vi "To Dynamic Signal.vi"(8 "error in (no error)":errorcluster, 11 "Software Lock-in in":refnum<class "Software Lock-in.lvclass">) -> (0 "error out":errorcluster, 1 "Channel names":string[](array[string]), 2 "Signal":dynamicdata(graph), 3 "Software Lock-in out":refnum<class "Software Lock-in.lvclass">, 4 "Time axis":dbl[](array[numeric]), 5 "dt":dbl)   [LabVIEW 2020, in "Software Lock-in.lvclass"]
uses:
  Software Lock-in.lvclass
  C:/GitHub/NHMFL_Core/Libraries/SoftwareLockin/Lock-in Detector/Lock-in Detector.lvclass
  Lock-in Detector/Lock-in Detector.lvclass/Lock-in Detector.ctl
  Software Lock-in.lvclass/Software Lock-in.ctl
  Lock-in Detector/Read Harmonic.vi
  Lock-in Detector/Read Decimation factor.vi
  Lock-in Detector/Read Sample rate.vi
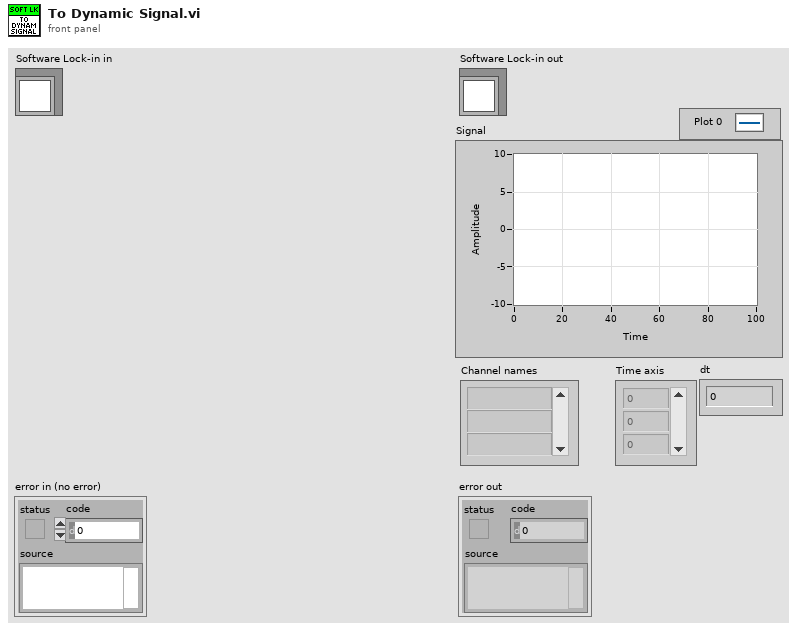
[diagram p1: front panel]
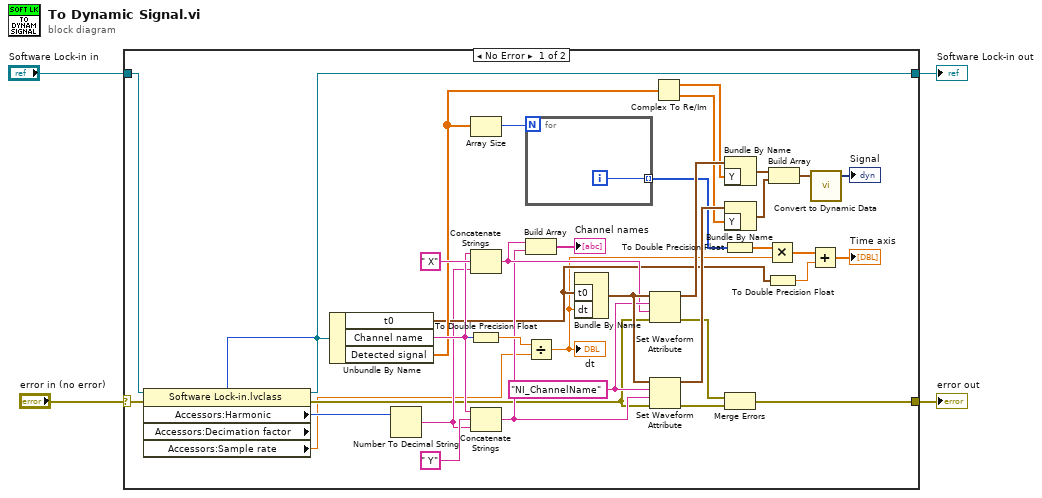
[diagram p0: block diagram]
diagram:
  n1 = case shown="No Error" "error in (no error)" {
    selector: "error in (no error)" -> [w25 w44]
    tunnel: [w24 w44] -> w3
    tunnel: [w8 w43] -> w1
    tunnel: "Software Lock-in in" -> [w9 w43]
    frame No Error {
      w38 = "NI_ChannelName" ("Channel Name")
      n2 = property class="Software Lock-in.lvclass"(reference=w9, error in=w25) -> (reference out=w8:refnum<class "Software Lock-in.lvclass">, error out=w10:errorcluster, "Accessors:Harmonic"=w7:i32, "Accessors:Decimation factor"=w6:i32, "Accessors:Sample rate"=w5:dbl)
      n3 = Unbundle By Name(w8) -> ("t0"=w15:timestamp, "Channel name"=w36:string, "Detected signal"=w20:cdb[])
      n4 = Number To Decimal String(number=w7) -> (decimal integer string=w11:string)  [unwired: 1 in]
      n5 = Array Size(array=w20) -> (size(s)=w19:i32)
      n6 = Concatenate Strings(w36, " X" ("string"), w11) -> (w23:string)
      n7 = To Double Precision Float(number=w6) -> (double precision float=w41:dbl)
      n8 = Concatenate Strings(w36, " Y" ("string"), w11) -> (w22:string)
      n9 = for {
        N: w19 -> [_]
        tunnel: [w42] -> w18 mode=indexing
        i -> [w42]
      }
      n10 = Build Array(w23, w22) -> (→"Channel names":string[])
      n11 = Divide(x=w41, y=w5) -> (x/y=w12:dbl)
      "dt" <- w12
      n12 = Bundle By Name("t0"=w15, "dt"=w12) -> (w39:waveform(dbl))  [unwired: 1 in]
      n13 = Set Waveform Attribute(4:w10, 5:w23, 6:w38, 7:w39) -> (0:w27:errorcluster, 3:w35:waveform(dbl))  [unwired: 1 out]
      n14 = Set Waveform Attribute(4:w10, 5:w22, 6:w38, 7:w39) -> (0:w26:errorcluster, 3:w33:waveform(dbl))  [unwired: 1 out]
      n15 = Complex To Re/Im(x + iy=w20) -> (x=w34:dbl[], y=w32:dbl[])
      n16 = Bundle By Name(cluster=w35, "Y"=w34) -> (w31:waveform(dbl))
      n17 = Bundle By Name(cluster=w33, "Y"=w32) -> (w30:waveform(dbl))
      n18 = To Double Precision Float(number=w18) -> (double precision float=w17:dbl[])
      n19 = Merge Errors(w27, w26) -> (w24:errorcluster)
      n20 = Multiply(x=w17, y=w12) -> (x*y=w16:dbl[])
      n21 = To Double Precision Float(number=w15) -> (double precision float=w14:dbl)
      n22 = Build Array(w31, w30) -> (w29:waveform(dbl)[])
      n23 = Add(x=w16, y=w14) -> (x+y=→"Time axis":dbl[])
      n24 = call "Convert to Dynamic Data"("Array of Waveforms"=w29) -> ("Dynamic Data Type"=→"Signal":dynamicdata)  [unwired: 3 in]
    }
    frame Error {
    }
  }
  "error out" <- w3
  "Software Lock-in out" <- w1
